vi "Set UI Loop References.vi"(7 "UI Data in":T1={"SR Display List"=[], "Filter Cluster"={"Show Resolved"=TRUE, "Show Potentially Resolved"=TRUE, "Show Passoffs"=TRUE, "Show In Collab"=TRUE}, "Exit"=refnum, "Main VI"=refnum, "Sorting"=enum."SR Status", "SR Display List"=refnum} {"SR Display List"."Creation Date" format="%<%x>T"; "SR Display List"."Last Updated" format="%<%x>T"}, 8 "error in (no error)":errorcluster, 11 "call chain":string[](array[string])) -> (0 "error out":errorcluster, 1 "UI Data out":T1 {"SR Display List"."Creation Date" format="%<%x>T"; "SR Display List"."Last Updated" format="%<%x>T"}, 3 "VI reference out":refnum<vi>)   [LabVIEW 2018]
uses:
  Type Defs/UI Loop Data.ctl
  Type Defs/SR Cluster.ctl
  Type Defs/SR Status.ctl
  Type Defs/Filter Cluster.ctl
  Type Defs/Sorting Methods.ctl
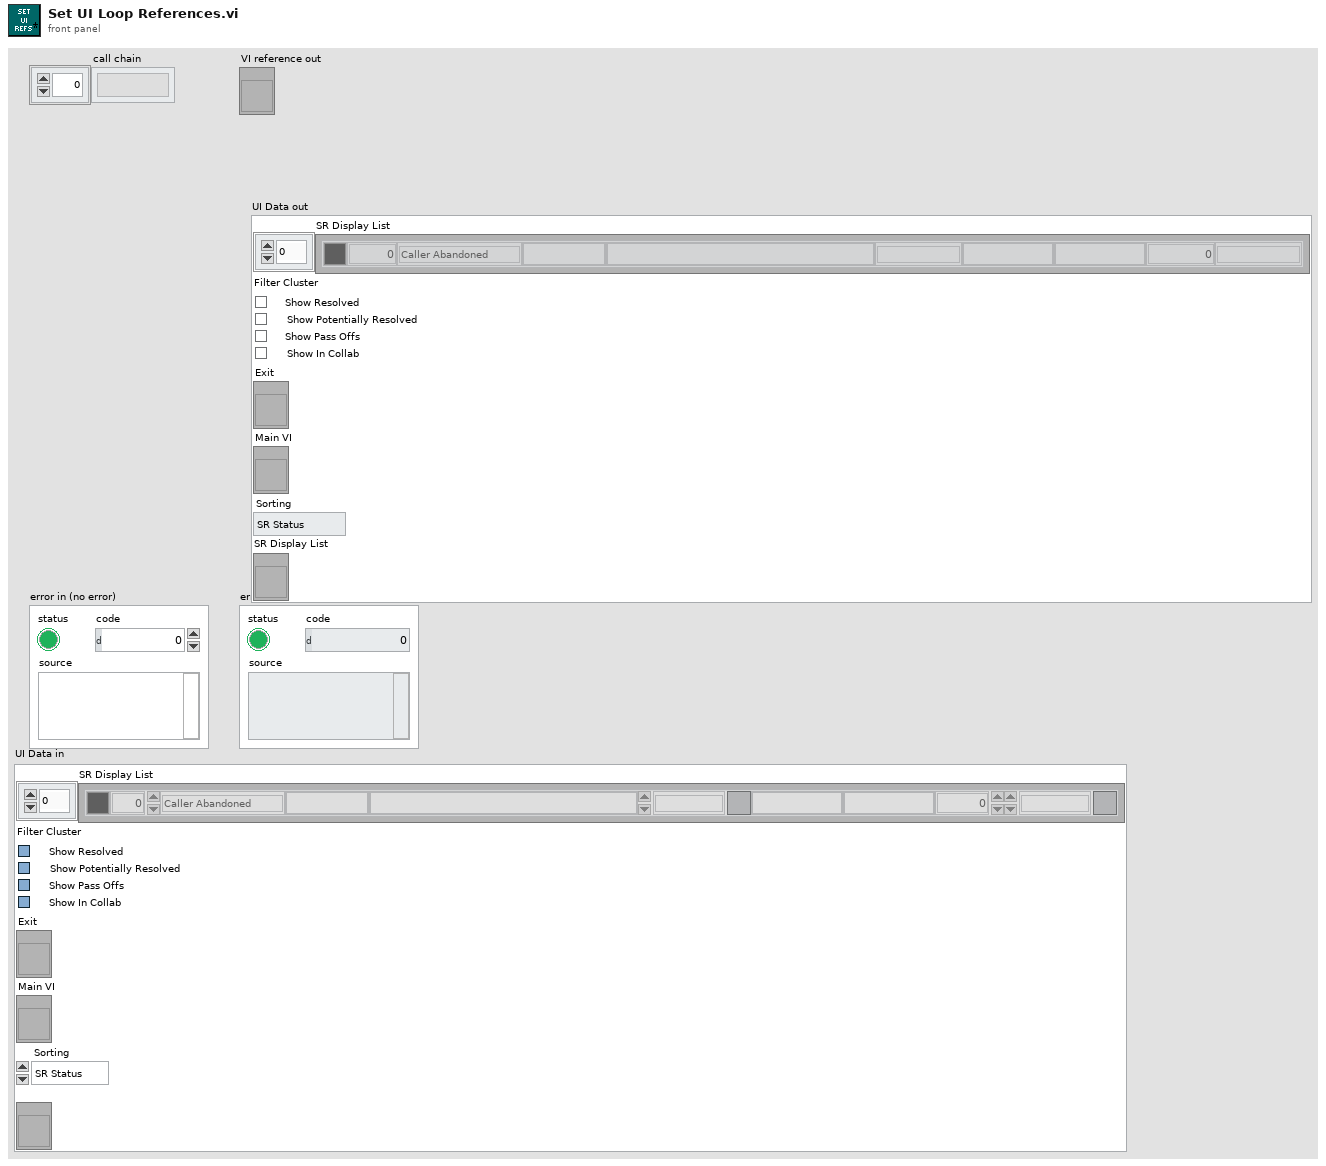
[diagram p1: front panel]
types:
  T1 = typedef "UI Loop Data.ctl" = cluster{"SR Display List":T2[], "Filter Cluster":T4, "Exit":refnum<vi>, "Main VI":refnum<vi>, "Sorting":T5, "SR Display List":refnum<vi>}
  T2 = typedef "SR Cluster.ctl" = cluster{"Color":u32, "SR Number":i32, "SR Status":T3, "Name":string, "Summary":string, "Last Updated":timestamp, "SR Type":string, "Service Level":string, "Days Open":dbl, "Creation Date":timestamp}
  T3 = typedef "SR Status.ctl" = enum16{"Caller Abandoned", "Created in Error", "Expired", "Forum Resolved AE", "Forum Resolved Customer", "IN WORK", "IN WORK Collab with AES", "IN WORK Collab with PSE", "IN WORK Collab with SE", "IN WORK Customer Added Note", "IN WORK Escalation", "IN WORK Wait on Customer", "Open", "Potentially Resolved", "Presumed Resolved", "RMA Approved for Return", "Resolved", "Passed Off"}
  T4 = typedef "Filter Cluster.ctl" = cluster{"Show Resolved":bool, "Show Potentially Resolved":bool, "Show Passoffs":bool, "Show In Collab":bool}
  T5 = typedef "Sorting Methods.ctl" = enum16{"SR Status", "Most Recent", "SR Type", "SR Number"}
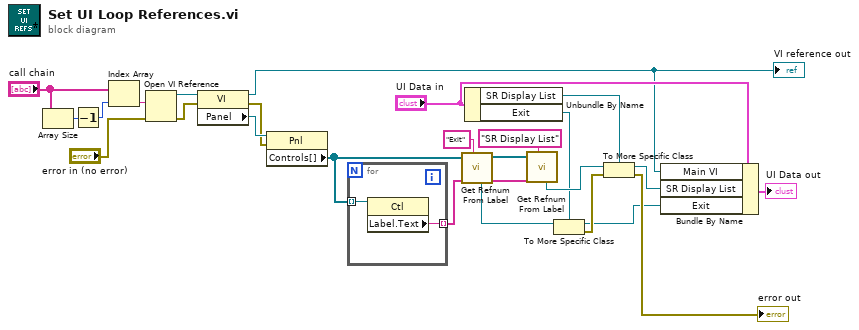
[diagram p0: block diagram]
diagram:
  n1 = Array Size(array="call chain") -> (size(s)=w5:i32)
  n2 = Decrement(x=w5) -> (x-1=w6:i32)
  n3 = Index Array(array="call chain", index=w6) -> (element=w7:string)
  n4 = Open VI Reference(vi path=w7, error in (no error)="error in (no error)") -> (vi reference=w26:refnum<vi>, error out=w21:errorcluster)  [unwired: 4 in]
  n5 = property class="VI"(reference=w26, error in=w21) -> (reference out=w3:refnum<vi>, error out=w22:errorcluster, "Panel"=w23:refnum<vi>)
  "VI reference out" <- w3
  n6 = property class="Pnl"(reference=w23, error in=w22) -> ("Controls[]"=w9:refnum<vi>[])  [unwired: 2 out]
  n7 = for {
    tunnel: w9 -> [w28] mode=indexing
    tunnel: [w27] -> w10 mode=indexing
    n8 = property class="Ctl"(reference=w28) -> ("Label.Text"=w27:string)  [unwired: 1 in, 2 out]
  }
  n9 = call "Get Refnum From Label.vi"("label"="Exit", "label array in"=w10, "controls[] in"=w9) -> ("label array out"=w12:string[], "controls[] out"=w11:refnum<vi>[], "refnum out"=w15:refnum<vi>)  [unwired: 6 in]
  n10 = Unbundle By Name("UI Data in") -> ("SR Display List"=w2:refnum<vi>, "Exit"=w14:refnum<vi>)
  n11 = call "Get Refnum From Label.vi"("label"="SR Display List", "label array in"=w12, "controls[] in"=w11) -> ("refnum out"=w19:refnum<vi>)  [unwired: 6 in, 2 out]
  n12 = To More Specific Class(target class=w14, reference=w15) -> (specific class reference=w13:refnum<vi>, error out=w17:errorcluster)  [unwired: 1 in]
  n13 = To More Specific Class(target class=w2, reference=w19, error in=w17) -> (specific class reference=w1:refnum<vi>, error out=→"error out":errorcluster)
  n14 = Bundle By Name(cluster="UI Data in", "Main VI"=w3, "SR Display List"=w1, "Exit"=w13) -> (→"UI Data out":T1)
